vi "2020_day08 (subVI run check).vi"(11 "lines":string[](array[string])) -> (1 "Reached End of Instruction List?":bool, 3 "ACC":i32)   [LabVIEW 2021]
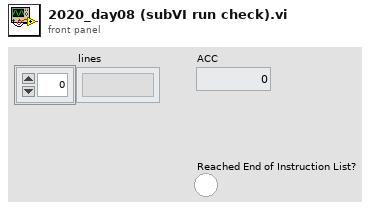
[diagram p1: front panel]
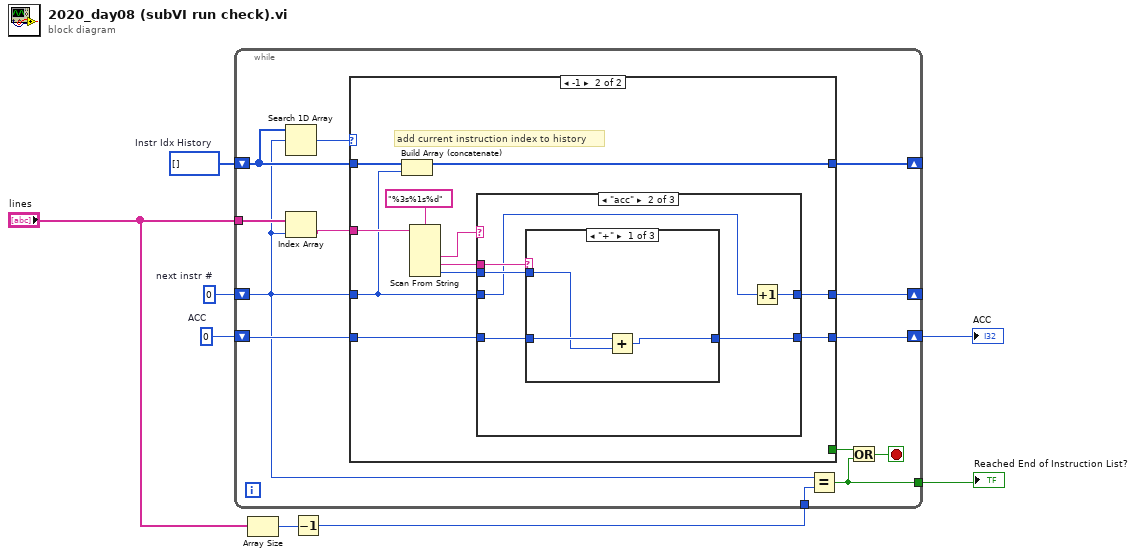
[diagram p0: block diagram]
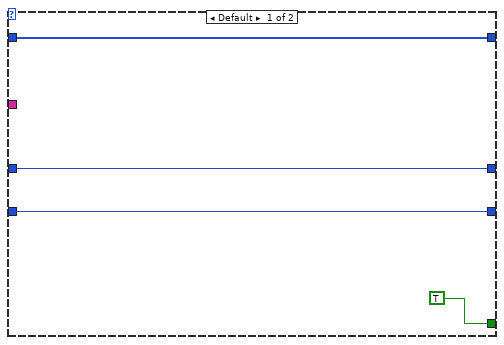
[diagram p2: hidden frame]
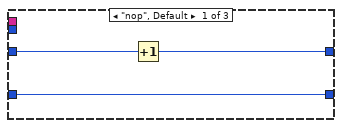
[diagram p3: hidden frame]
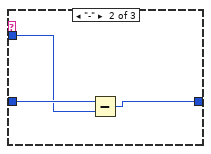
[diagram p4: hidden frame]
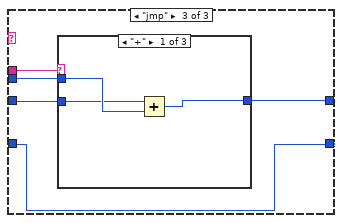
[diagram p6: hidden frame]
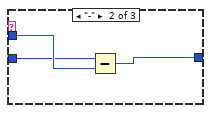
[diagram p7: hidden frame]
diagram:
  w3 = 0  # ACC
  w2 = 0  # next instr #
  w1 = i32[] []  # Instr Idx History
  n1 = Array Size(array="lines") -> (size(s)=w6:i32)
  n2 = Decrement(x=w6) -> (x-1=w7:i32)
  n3 = while {
    tunnel: "lines" -> [w21]
    shift-right: [w14] -> _
    shift-left: w1 -> [w20]
    shift-right: [w12] -> _
    shift-left: w2 -> [w11]
    shift-right: [w17] -> w4
    shift-left: w3 -> [w16]
    tunnel: w7 -> [w13]
    tunnel: [w9] -> w8
    stop <- w10 stop-if-true
    n4 = Search 1D Array(1D array=w20, element=w11) -> (index of element=w19:i32)  [unwired: 1 in]
    n5 = Index Array(array=w21, index=w11) -> (element=w18:string)
    n6 = case shown="-1" w19 {
      tunnel: w20 -> [w22 w36]
      tunnel: w11 -> [w25 w26]
      tunnel: [w25 w27] -> w12
      tunnel: w18 -> [_ w34]
      tunnel: [w24 w31] -> w17
      tunnel: w16 -> [w24 w30]
      tunnel: [TRUE _] -> w15
      tunnel: [w22 w35] -> w14
      frame Default {
      }
      frame -1 {
        # "add current instruction index to history"
        n7 = Build Array (concatenate)(w36, w26) -> (w35:i32[])
        n8 = Scan From String(format string="%3s%1s%d", input string=w34) -> (output 1=w32:string, output 2=w29:string, output 3=w28:i32)  [unwired: 5 in, 3 out]
        n9 = case shown="\"acc\"" w32 {
          tunnel: [w39 w43 w53] -> w31
          tunnel: w30 -> [w39 w42 w53]
          tunnel: w29 -> [_ w45 w57]
          tunnel: w28 -> [_ w44 w56]
          tunnel: [w37 w40 w54] -> w27
          tunnel: w26 -> [w38 w41 w55]
          frame "nop", Default {
            n10 = Increment(x=w38) -> (x+1=w37:i32)
          }
          frame "acc" {
            n11 = case shown="\"+\"" w45 {
              tunnel: w44 -> [w46 w49 _]
              tunnel: [w47 w50 w52] -> w43
              tunnel: w42 -> [w48 w51 w52]
              frame "+" {
                n12 = Add(x=w48, y=w46) -> (x+y=w47:i32)
              }
              frame "-" {
                n13 = Subtract(x=w51, y=w49) -> (x-y=w50:i32)
              }
              frame Default {
              }
            }
            n14 = Increment(x=w41) -> (x+1=w40:i32)
          }
          frame "jmp" {
            n15 = case shown="\"+\"" w57 {
              tunnel: w56 -> [w60 w63 _]
              tunnel: w55 -> [w59 w61 w64]
              tunnel: [w58 w62 w64] -> w54
              frame "+" {
                n16 = Add(x=w59, y=w60) -> (x+y=w58:i32)
              }
              frame "-" {
                n17 = Subtract(x=w61, y=w63) -> (x-y=w62:i32)
              }
              frame Default {
              }
            }
          }
        }
      }
    }
    n18 = Equal?(x=w11, y=w13) -> (x = y?=w9:bool)
    n19 = Or(x=w15, y=w9) -> (x .or. y?=w10:bool)
  }
  "Reached End of Instruction List?" <- w8
  "ACC" <- w4
